vi "Shooter Arm.vi"(8 "Boolean 2":bool, 9 "Boolean":bool, 11 "Arm Ref":string) -> ()   [LabVIEW 2014]
uses:
  <vilib>/Rock Robotics/WPI/Solenoid/WPI_SolenoidValue.ctl
  <vilib>/Rock Robotics/WPI/Relay/WPI_RelayValue.ctl
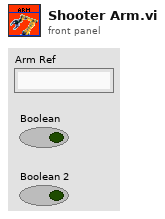
[diagram p1: front panel]
types:
  T1 = typedef "WPI_RelayValue.ctl" = enum16{"Off", "On", "Forward", "Reverse"}
  T2 = typedef "WPI_SolenoidValue.ctl" = enum16{"Off", "On", "Forward", "Reverse"}
  T3 = typedef "WPI_RelayDevRef.ctl" = cluster{"DevStatus":errorcluster, "Relay Channel":T4, "Controller":T5, "Relay Direction":T6}
  T4 = typedef "FPGA_DIORelayChannel.ctl" = enum8{"Relay 0", "Relay 1", "Relay 2", "Relay 3", "Invalid"}
  T5 = typedef "FPGA_TypedefDigitalModule.ctl" = enum16{"Controller 1"}
  T6 = typedef "WPI_RelayDirection.ctl" = enum16{"Both directions", "Forward only", "Reverse only"}
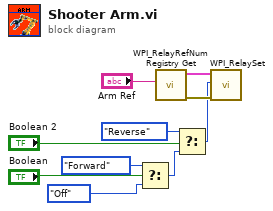
[diagram p0: block diagram]
diagram:
  n1 = Select(t=WPI_SolenoidValue."Forward" ("Value"), s="Boolean", f=WPI_RelayValue."Off" ("RelayValue")) -> (s? t:f=w2:T1)
  n2 = call <vilib>:"WPI_RelayRefNum Registry Get.vi"("refnum name"="Arm Ref") -> ("error out"=w7:errorcluster, "RelayDevRef"=w6:T3)  [unwired: 9 in]
  n3 = Select(t=WPI_SolenoidValue."Reverse" ("Value"), s="Boolean 2", f=w2) -> (s? t:f=w1:T1)
  n4 = call <vilib>:"WPI_RelaySet.vi"("error in (no error)"=w7, "RelayValue"=w1, "RelayDevRef"=w6) -> ()  [unwired: 7 in, 2 out]
